vi "main_old.vi"() -> ()   [LabVIEW 2018]
uses:
  Control 12.ctl
  <vilib>/Instr/_visa.llb/VISA Configure Serial Port (Instr).vi
panel:
  in  "Tab Control":T1(tab)
  out "Temperatura (ºC)":dbl(slide) scale=0.0..50.0 scale format="%#.2f"
  out "Acceleròmetre":cluster{dbl, dbl, dbl}(graph)={-1477.92, 1162.76, -1186.5} caption="Waveform Chart - Dark"
  out "Giroscòpi":cluster{dbl, dbl, dbl}(graph)={-1477.92, 1162.76, -1186.5} caption="Waveform Chart - Dark"
  out "Magnetometre":cluster{dbl, dbl, dbl}(graph)={-4031.37, -986.16, -4204.69} caption="Waveform Chart - Dark"
  out "All Data":string
  in  "STOP 2":bool
  in  "START 2":bool
  in  "CONFIG SEL":bool
  in  "MOT SEL 3":bool
  out "Bobina 3":bool
  out "Bobina 2":bool
  out "Bobina 1":bool
  out "Motor":cluster{"Data Out":dbl, "Data Out":dbl}(graph) caption="Waveform Chart - Dark"
  in  "START 3":bool
  in  "STOP 3":bool
  in  "CONFIG SEL   2":bool
  in  "IMU SEL  3":bool
  in  "Configuracions de VISA (UART)":T3={"stop bits (10: 1 bit)"=10, "baud rate "=115200, "parity (0:none)"=enum."None", "data bits (8)"=8, "Enable Termination\nChar"=TRUE, "termination char\n(0xA = '\\n' = LF) "=0, "Timeout "=10000, "VISA"="COM4"} {"termination char\n(0xA = '\\n' = LF)" format="%.0x"; "data bits (8)" min=5 max=8 step=1; "stop bits (10: 1 bit)" items=["1.0"=10, "1.5"=15, "2.0"=20]}
  in  "STOP":bool
  in  "START 3":bool
  in  "MOT SEL":bool
  in  "IMU SEL":bool
  in  "Debug SEL 3":bool
  out "Motor DataString":string
  out "All Data":string
  out "Error out":errorcluster
  in  "STOP 4":bool
  in  "START 4":bool
  out "VISA Buffer count":u32
  in  "MOCK CTRL":bool
  in  "Write a mock string":string=":0,0,0;0,0,0;0,0,0;0,0;"
  out "read buffer":string
  in  "Default":bool
  in  "CONFIG SEL   3":bool
  in  "MOT SEL 2":bool
  in  "IMU SEL  2":bool
  # "Angle"
  # "Fase"
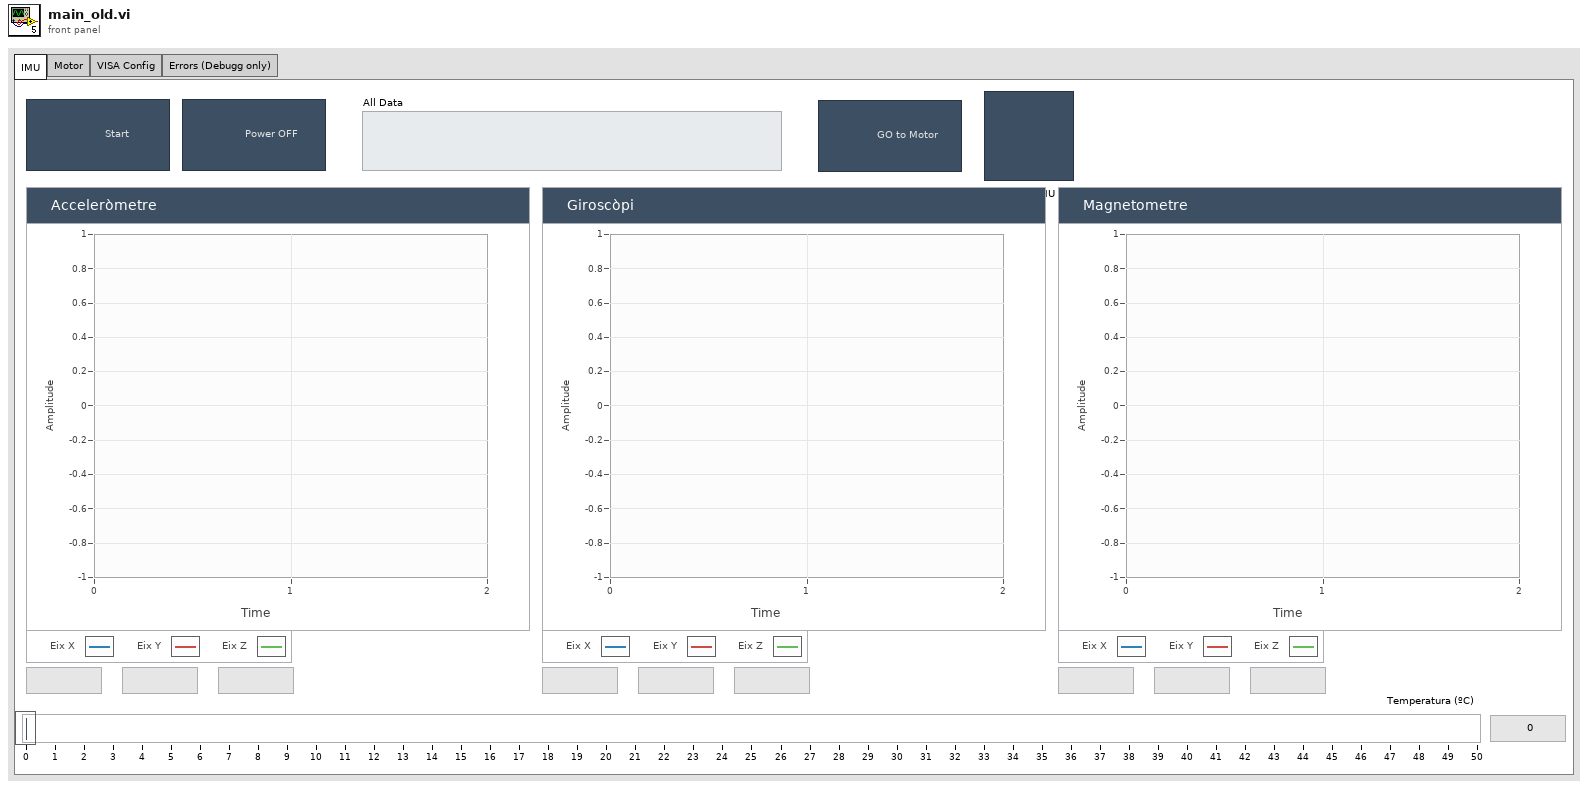
[diagram p1: front panel]
types:
  T1 = enum32{"IMU", "Motor", "VISA Config", "Errors (Debugg only)"}
  T2 = typedef "Control 12.ctl" = refnum<visa-resource-name>
  T3 = cluster{"stop bits (10: 1 bit)":u16, "baud rate ":u32, "parity (0:none)":enum16{"None", "Odd", "Even", "Mark", "Space"}, "data bits (8)":u16, "Enable Termination\nChar":bool, "termination char\n(0xA = '\\n' = LF) ":u8, "Timeout ":u32, "VISA":T2}
  T4 = cluster{"ShiftReg Right":cluster{"shift register right":string, "shift register right":string, "shift register right":string}, "ShiftReg Right":cluster{"shift register right":string, "shift register right":string, "shift register right":string}, "ShiftReg Right":cluster{"shift register right":string, "shift register right":string, "shift register right":string}, "ShiftReg RIGHT":cluster{"shift register right":string, "shift register right 2":string, "shift register right 3":string}, "read buffer":string}
  T5 = cluster{"shift register right":string, "shift register right":string, "shift register right":string}
  T6 = cluster{"shift register right":string, "shift register right 2":string, "shift register right 3":string}
  T7 = cluster{"Angle (graus)":dbl, "Fase (#bobina)":dbl, "Temp":dbl}
  T8 = cluster{"ShiftReg Right":cluster{"shift register right":string, "shift register right":string, "shift register right":string}, "ShiftReg Right":cluster{"shift register right":string, "shift register right":string, "shift register right":string}, "ShiftReg Right":cluster{"shift register right":string, "shift register right":string, "shift register right":string}, "ShiftReg RIGHT":cluster{"shift register right":string, "shift register right 2":string, "shift register right 3":string}, "Write a mock string":string}
  T9 = cluster{"Angle (graus)":dbl, "Fase (#bobina)":dbl}
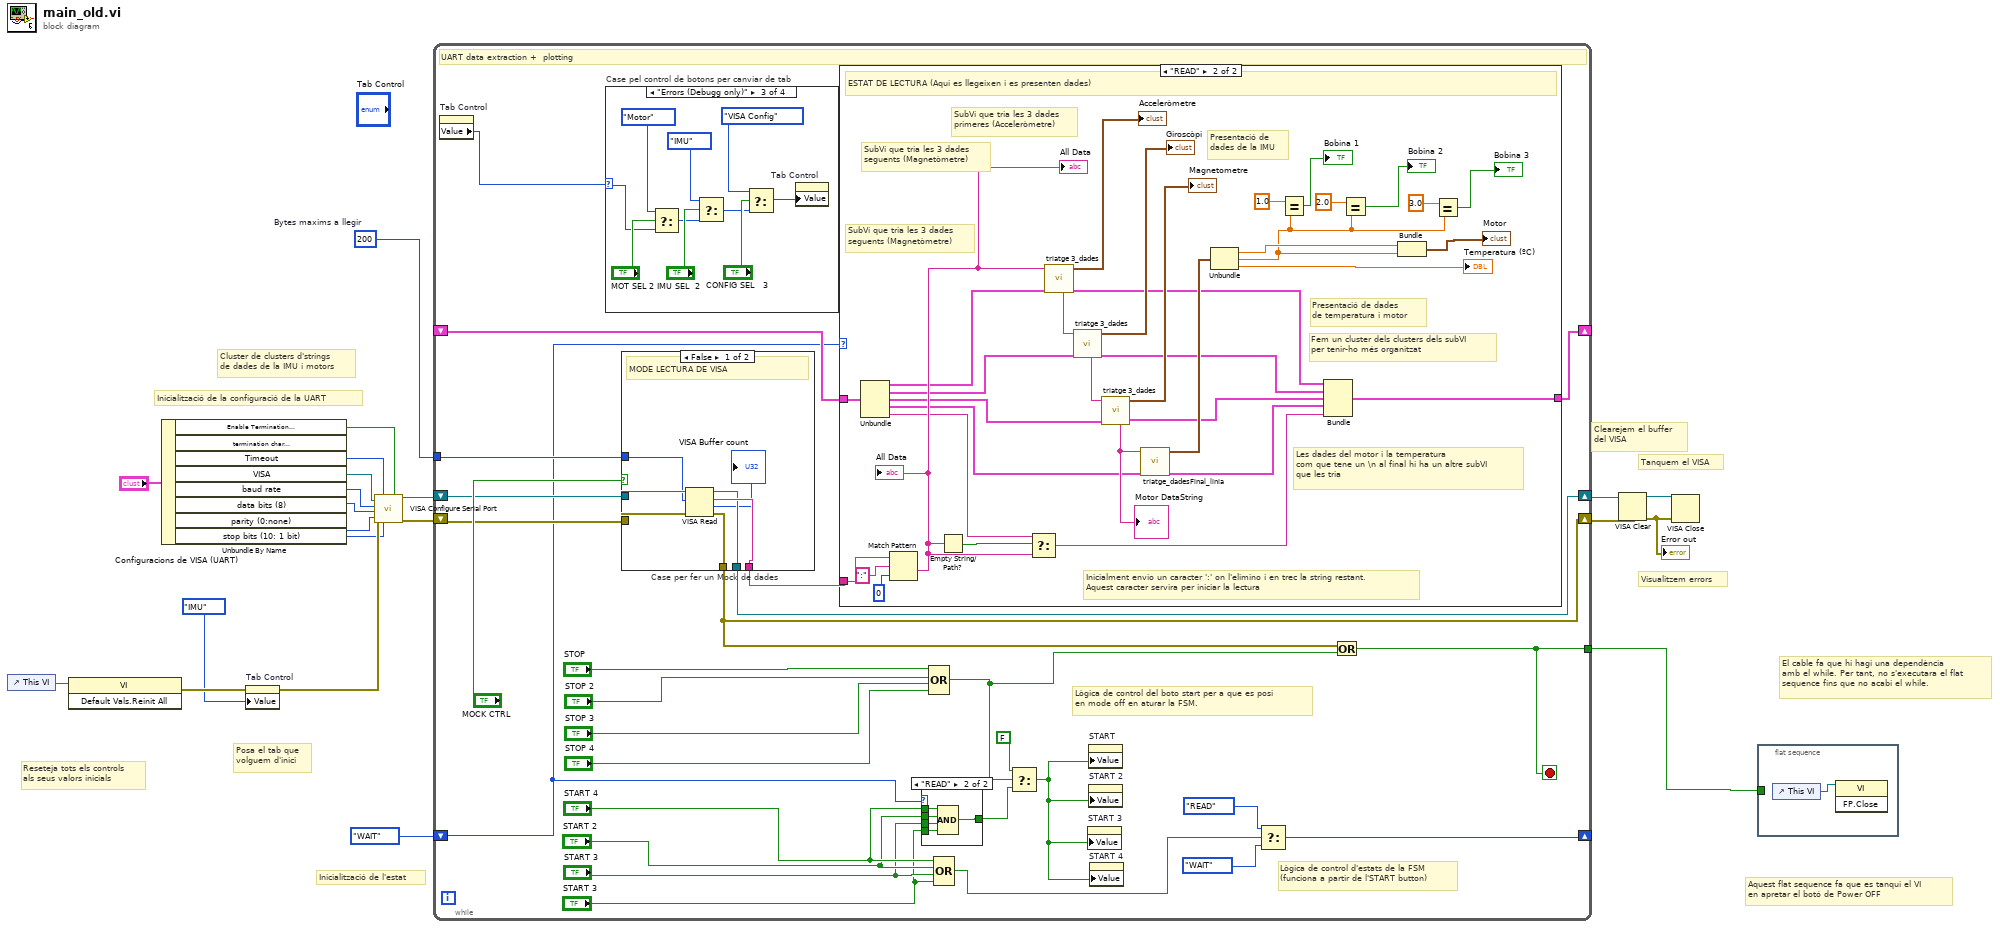
[diagram p0: block diagram]
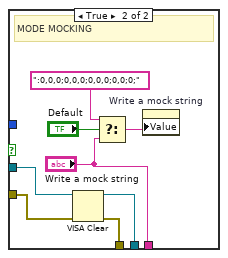
[diagram p2: hidden frame]
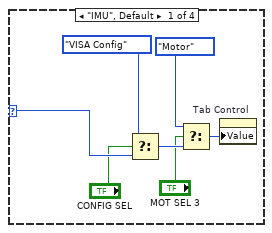
[diagram p3: hidden frame]
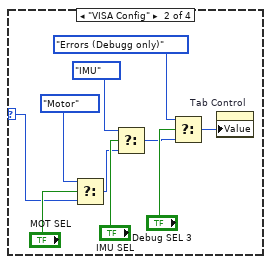
[diagram p4: hidden frame]
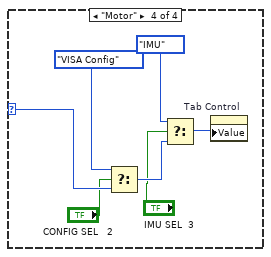
[diagram p5: hidden frame]
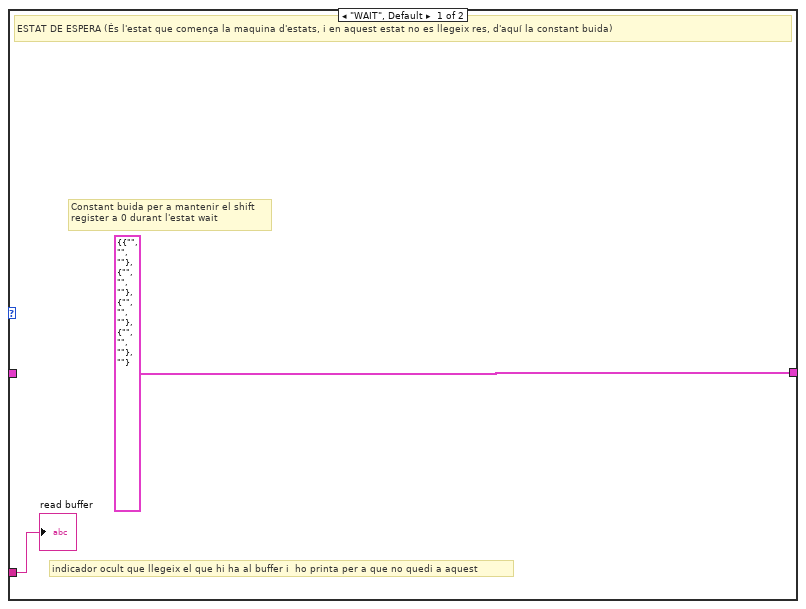
[diagram p6: hidden frame]
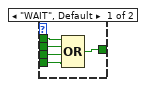
[diagram p7: hidden frame]
diagram:
  w13 = u32 200  # Bytes maxims a llegir
  # "Inicialització de l'estat"
  # "Visualitzem errors"
  # "Clearejem el buffer\ndel VISA"
  # "Cluster de clusters d'strings\nde dades de la IMU i motors"
  # "Tanquem el VISA"
  # "Inicialització de la configuració de la UART"
  # "Posa el tab que\nvolguem d'inici"
  # "Reseteja tots els controls \nals seus valors inicials"
  # "Aquest flat sequence fa que es tanqui el VI\nen apretar el botó de Power OFF"
  # "El cable fa que hi hagi una dependència\namb el while. Per tant, no s'executara el flat\nsequence fins que no acabi el while."
  n1 = control-ref of="This VI"() -> (w20:refnum<vi>)
  n2 = invoke class="VI" method="Default Vals.Reinit All"(reference=w20) -> (error out=w19:errorcluster)  [unwired: 2 in, 2 out]
  n3 = Unbundle By Name("Configuracions de VISA (UART)") -> ("Enable Termination\nChar"=w8:bool, "Timeout"=w7:u32, "VISA"=w6:T2, "baud rate"=w5:u32, "data bits (8)"=w4:u16, "parity (0:none)"=w3:enum16{"None", "Odd", "Even", "Mark", "Space"}, "stop bits (10: 1 bit)"=w2:u16)  [unwired: 1 out]
  n4 = property on="Tab Control" class="TabCtl (strict)"(error in=w19, "Value"=T1."IMU" ("t")) -> (error out=w18:errorcluster)  [unwired: 1 in, 1 out]
  n5 = call-poly "VISA Configure Serial Port"("VISA resource name"=w6, "timeout (10sec)"=w7, "Enable Termination\nChar (T)"=w8, "baud rate (9600)"=w5, "data bits (8)"=w4, "parity (0:none)"=w3, "error in (no error)"=w18, "stop bits (10: 1 bit)"=w2) -> ("VISA resource name out"=w14:refnum<visa-resource-name>, "error out"=w16:errorcluster)  [unwired: 6 in]
  n6 = while {
    shift-right: [w23] -> _
    shift-left: enum16{"WAIT", "READ", ""}."WAIT" -> [w25]
    shift-right: [w49] -> w11
    shift-left: w16 -> [w29]
    shift-right: [w42] -> w15
    shift-left: w14 -> [w30]
    shift-right: [w33] -> _
    shift-left: _ -> [w27]
    tunnel: [w22] -> w21
    tunnel: w13 -> [w28]
    stop <- w22 stop-if-true
    # "Lògica de control d'estats de la FSM\n(funciona a partir de l'START button)"
    # "Lògica de control del boto start per a que es posi \nen mode off en aturar la FSM."
    # "UART data extraction +  plotting"
    n7 = property on="Tab Control" class="TabCtl (strict)"() -> ("Value"=w26:T1)  [unwired: 2 in, 2 out]
    n8 = case "Case pel control de botons per canviar de tab" shown="\"Errors (Debugg only)\"" w26 {
      selector: w26 -> [w71 w74 w83 w97]
      frame "IMU", Default {
        n9 = Select(t=T1."VISA Config", s="CONFIG SEL", f=w71) -> (s? t:f=w67:T1)
        n10 = Select(t=T1."Motor", s="MOT SEL 3", f=w67) -> (s? t:f=w68:T1)
        n11 = property on="Tab Control" class="TabCtl (strict)"("Value"=w68) -> ()  [unwired: 2 in, 2 out]
      }
      frame "VISA Config" {
        n12 = Select(t=T1."Motor", s="MOT SEL", f=w74) -> (s? t:f=w79:T1)
        n13 = Select(t=T1."IMU", s="IMU SEL", f=w79) -> (s? t:f=w73:T1)
        n14 = Select(t=T1."Errors (Debugg only)", s="Debug SEL 3", f=w73) -> (s? t:f=w72:T1)
        n15 = property on="Tab Control" class="TabCtl (strict)"("Value"=w72) -> ()  [unwired: 2 in, 2 out]
      }
      frame "Errors (Debugg only)" {
        n16 = Select(t=T1."Motor", s="MOT SEL 2", f=w83) -> (s? t:f=w86:T1)
        n17 = Select(t=T1."IMU", s="IMU SEL  2", f=w86) -> (s? t:f=w82:T1)
        n18 = Select(t=T1."VISA Config", s="CONFIG SEL   3", f=w82) -> (s? t:f=w90:T1)
        n19 = property on="Tab Control" class="TabCtl (strict)"("Value"=w90) -> ()  [unwired: 2 in, 2 out]
      }
      frame "Motor" {
        n20 = Select(t=T1."VISA Config", s="CONFIG SEL   2", f=w97) -> (s? t:f=w95:T1)
        n21 = Select(t=T1."IMU", s="IMU SEL  3", f=w95) -> (s? t:f=w96:T1)
        n22 = property on="Tab Control" class="TabCtl (strict)"("Value"=w96) -> ()  [unwired: 2 in, 2 out]
      }
    }
    n23 = case "Case per fer un Mock de dades" shown="False" "MOCK CTRL" {
      tunnel: [w56 "Write a mock string"] -> w31
      tunnel: [w55 w64] -> w49
      tunnel: [w54 w63] -> w42
      tunnel: w30 -> [w53 w58]
      tunnel: w29 -> [w52 w57]
      tunnel: w28 -> [w51 _]
      frame False {
        # "MODE LECTURA DE VISA"
        n24 = VISA Read(VISA resource name=w53, byte count=w51, error in (no error)=w52) -> (VISA resource name out=w54:refnum<visa-resource-name>, read buffer=w56:string, return count=→"VISA Buffer count":u32, error out=w55:errorcluster)
      }
      frame True {
        # "MODE MOCKING"
        n25 = VISA Clear(VISA resource name=w58, error in (no error)=w57) -> (VISA resource name out=w63:refnum<visa-resource-name>, error out=w64:errorcluster)
        n26 = Select(t=":0,0,0;0,0,0;0,0,0;0,0;0;" ("Write a mock string"), s="Default", f="Write a mock string") -> (s? t:f=w62:string)
        n27 = property on="Write a mock string" class="Str"("Value"=w62) -> ()  [unwired: 2 in, 2 out]
      }
    }
    n28 = case shown="\"READ\"" w25 {
      tunnel: w31 -> [w99 w101]
      tunnel: [T4 {"ShiftReg Right"={"shift register right"="", "shift register right"="", "shift register right"=""}, "ShiftReg Right"={"shift register right"="", "shift register right"="", "shift register right"=""}, "ShiftReg Right"={"shift register right"="", "shift register right"="", "shift register right"=""}, "ShiftReg RIGHT"={"shift register right"="", "shift register right 2"="", "shift register right 3"=""}, "read buffer"=""} w109] -> w33
      tunnel: w27 -> [_ w108]
      frame "WAIT", Default {
        # "Constant buida per a mantenir el shift\nregister a 0 durant l'estat wait"
        # "indicador ocult que llegeix el que hi ha al buffer i  ho printa per a que no quedi a aquest"
        # "ESTAT DE ESPERA (És l'estat que comença la maquina d'estats, i en aquest estat no es llegeix res, d'aquí la constant buida)"
        "read buffer" <- w99
      }
      frame "READ" {
        # "Inicialment envio un caracter ':' on l'elimino i en trec la string restant.\nAquest caracter servira per iniciar la lectura"
        # "Presentació de \ndades de la IMU"
        # "Presentació de dades\nde temperatura i motor"
        # "Fem un cluster dels clusters dels subVI\nper tenir-ho més organitzat"
        # "Les dades del motor i la temperatura \ncom que tene un \\n al final hi ha un altre subVI\nque les tria"
        # "SubVi que tria les 3 dades\nseguents (Magnetòmetre)"
        # "SubVi que tria les 3 dades\nseguents (Magnetòmetre)"
        # "SubVi que tria les 3 dades\nprimeres (Acceleròmetre)"
        # "ESTAT DE LECTURA (Aqui es llegeixen i es presenten dades)"
        n29 = Unbundle(w108) -> ("ShiftReg Right"=w107:T5, "ShiftReg Right"=w106:T5, "ShiftReg Right"=w105:T5, "ShiftReg RIGHT"=w104:T6, "Write a mock string"=w103:string)
        n30 = Match Pattern(string=w101, regular expression=":", offset (0)=0 ("t")) -> (after substring=w121:string)  [unwired: 3 out]
        "All Data" <- w121
        "All Data" <- w121
        n31 = Empty String/Path?(string/path=w121) -> (empty?=w132:bool)
        n32 = Select(t=w103, s=w132, f=w121) -> (s? t:f=w110:string)
        n33 = call "triatge 3_dades.vi"("Cluster - Borderless"=w107, "DataIN"=w121) -> ("ShiftReg Right"=w114:T5, "Acceleròmetre"=→"Acceleròmetre":cluster{dbl, dbl, dbl}, "String Out"=w124:string)  [unwired: 7 in]
        n34 = call "triatge 3_dades.vi"("Cluster - Borderless"=w106, "DataIN"=w124) -> ("ShiftReg Right"=w113:T5, "Acceleròmetre"=→"Giroscòpi":cluster{dbl, dbl, dbl}, "String Out"=w120:string)  [unwired: 7 in]
        n35 = call "triatge 3_dades.vi"("Cluster - Borderless"=w105, "DataIN"=w120) -> ("ShiftReg Right"=w112:T5, "Acceleròmetre"=→"Magnetometre":cluster{dbl, dbl, dbl}, "String Out"=w122:string)  [unwired: 7 in]
        "Motor DataString" <- w122
        n36 = call "triatge_dadesFinal_linia.vi"("ShiftReg LEFT"=w104, "String in"=w122) -> ("ShiftReg RIGHT"=w111:T6, "DADES"=w119:T7)  [unwired: 8 in]
        n37 = Unbundle(w119) -> ("Angle (graus)"=w118:dbl, "Fase (#bobina)"=w115:dbl, "Temp"=→"Temperatura (ºC)":dbl)
        n38 = Equal?(x=1.0, y=w115) -> (x = y?=→"Bobina 1":bool)
        n39 = Bundle("ShiftReg Right"=w114, "ShiftReg Right"=w113, "ShiftReg Right"=w112, "ShiftReg RIGHT"=w111, "Write a mock string"=w110) -> (w109:T8)  [unwired: 1 in]
        n40 = Equal?(x=2.0, y=w115) -> (x = y?=→"Bobina 2":bool)
        n41 = Bundle("Angle (graus)"=w118, "Fase (#bobina)"=w115) -> (→"Motor":T9)  [unwired: 1 in]
        n42 = Equal?(x=3.0, y=w115) -> (x = y?=→"Bobina 3":bool)
      }
    }
    n43 = case shown="\"READ\"" w25 {
      tunnel: "START 4" -> [w136 w144]
      tunnel: "START 2" -> [w139 w143]
      tunnel: "START 3" -> [w138 w142]
      tunnel: "START 3" -> [w137 w141]
      tunnel: [w135 w140] -> w24
      frame "WAIT", Default {
        n44 = Compound Arithmetic op=OR(w136, w139, w138, w137) -> (w135:bool)
      }
      frame "READ" {
        n45 = Compound Arithmetic op=AND(w144, w143, w142, w141) -> (w140:bool)
      }
    }
    n46 = Compound Arithmetic op=OR("STOP", "STOP 2", "STOP 3", "STOP 4") -> (w41:bool)
    n47 = Compound Arithmetic op=OR("START 4", "START 2", "START 3", "START 3") -> (w40:bool)
    n48 = Select(t=FALSE, s=w41, f=w24) -> (s? t:f=w35:bool)
    n49 = property on="START 3" class="Bool (strict)"("Value"=w35) -> ()  [unwired: 2 in, 2 out]
    n50 = property on="START" class="Bool (strict)"("Value"=w35) -> ()  [unwired: 2 in, 2 out]
    n51 = property on="START 2" class="Bool (strict)"("Value"=w35) -> ()  [unwired: 2 in, 2 out]
    n52 = property on="START 4" class="Bool (strict)"("Value"=w35) -> ()  [unwired: 2 in, 2 out]
    n53 = Select(t=enum16{"WAIT", "READ", ""}."READ", s=w40, f=enum16{"WAIT", "READ", ""}."WAIT") -> (s? t:f=w23:enum16{"WAIT", "READ", ""})
    n54 = Or(x=w49, y=w41) -> (x .or. y?=w22:bool)
  }
  n55 = VISA Clear(VISA resource name=w15, error in (no error)=w11) -> (VISA resource name out=w12:refnum<visa-resource-name>, error out=w10:errorcluster)
  "Error out" <- w10
  n56 = VISA Close(VISA resource name=w12, error in (no error)=w10) -> ()  [unwired: 1 out]
  n57 = flat-sequence {
    tunnel: w21 -> [_]
    frame #0 {
      n58 = control-ref of="This VI"() -> (w145:refnum<vi>)
      n59 = invoke class="VI" method="FP.Close"(reference=w145) -> ()  [unwired: 2 in, 3 out]
    }
  }
